vi "active_.vi"(2 "reference":refnum<vi>, 3 "error in (no error)":errorcluster) -> (6 "Active ON?":bool, 7 "error out":errorcluster)   [LabVIEW 2024]
uses:
  global/active_on_.vi
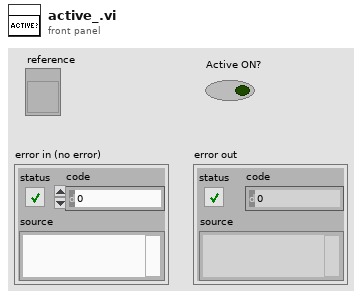
[diagram p1: front panel]
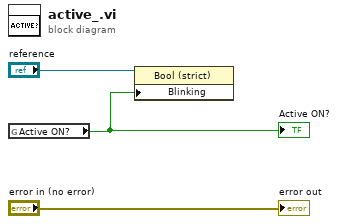
[diagram p0: block diagram]
diagram:
  n1 = global read "active_on_.vi" "Active ON?"() -> (w3:bool)
  "Active ON?" <- w3
  n2 = property class="Bool (strict)"(reference="reference", "Blinking"=w3) -> ()  [unwired: 1 in, 2 out]
  "error out" <- "error in (no error)"
